vi "cDAQ_Read.vi"(8 "error in":errorcluster, 9 "Prev Temp":dbl format="%0.2f", 10 "DAQ/Control":u16(ring) items=["DAQ", "Control"], 11 "DataCluster":T1={"Core"={"Current VI Reference"=refnum, "Close Panel on Exit?"=FALSE, "Exit"=FALSE}, "Connections"={"cDAQ Therm"={"Task"="", "Connected"=FALSE, "Active"=FALSE}, "cDAQ Voltage"={"Task"="", "Connected"=FALSE, "Active"=FALSE}, "Camera"={"Session"="", "Connected"=FALSE, "Active"=FALSE}}, "Data Acquisition"={"Setup"={"Label"="", "Operator"="", "Notes"="", "TempGrad"=1.0, "TargetTemp"=1.0, "Sample Volume"=1.0}, "Camera"={"Image"=refnum, "Save Image"=refnum, "Image Frequency"=20}, "Thermistor"={"Sample Size"=1, "Calibration"={"B0.100"=[], "R25"=[], "c"=[], "State"=[], "V_S"=5.0, "R_S"=100.0}, "Timing Mode"=14713}, "Partition"={"Data"=[], "Cell Label"="", "Cell Color"=0, "Height"=10, "Width"=16, "Grid"=[]}, "Queue"={"Size"=1, "Queue"=refnum}, "Sample Rate"=1, "Active"=FALSE, "Ready"=FALSE, "Graph Mode"=0}, "Control"={"Sample Rate"=1, "PID gains"={"proportional gain (Kc)"=1.0, "integral time (Ti, min)"=0.01, "derivative time (Td, min)"=0.0}}} {"Control"."PID gains"."derivative time (Td, min)" format="%.3f"; "Control"."PID gains"."integral time (Ti, min)" format="%.3f"; "Control"."PID gains"."proportional gain (Kc)" format="%.3f"; "Control"."Sample Rate" min=1 max=20 step=1 format="%.0f Samples/sec"; "Data Acquisition"."Graph Mode" items=["Average Temperature", "Individual Temperatures"]; "Data Acquisition"."Thermistor"."Timing Mode" items=["Automatic"=16097, "High Resolution"=10195, "High Speed"=14712, "Best 50 Hz Rejection"=14713, "Best 60 Hz Rejection"=14714, "Custom"=10137]; "Data Acquisition"."Thermistor"."Calibration"."R_S" min=0.1 max=1000.0 format="%#_g kOhm"; "Data Acquisition"."Thermistor"."Calibration"."V_S" min=5.0 max=48.0 format="%#_g V"; "Data Acquisition"."Thermistor"."Calibration"."R25" min=0.1 max=1000.0 format="%#_g kOhm"; "Data Acquisition"."Thermistor"."Calibration"."B0.100" min=100.0 max=10000.0 format="%#_g K"; "Data Acquisition"."Thermistor"."Sample Size" min=1 max=200; "Data Acquisition"."Sample Rate" min=20 max=240 format="%.0f samples/min"; "Data Acquisition"."Queue"."Size" min=1 max=200; "Data Acquisition"."Camera"."Image Frequency" min=1 max=60 step=1; "Data Acquisition"."Setup"."Sample Volume" min=0.0 max=500.0 format="%#_g µL"; "Data Acquisition"."Setup"."TargetTemp" min=-40.0 max=40.0 step=0.5 format="%#_g °C"; "Data Acquisition"."Setup"."TempGrad" min=-100.0 max=100.0 step=0.1 format="%#_g °C/min"}) -> (0 "Temp Gradient":dbl, 1 "Mean Temperature":dbl format="%0.2f", 2 "Temperature Readings":dbl[](array[numeric]), 3 "Voltage Readings":dbl[](array[numeric]), 4 "error out":errorcluster, 5 "valid sample?":bool)   [LabVIEW 2020]
uses:
  DataCluster.ctl
  <vilib>/userdefined/High Color/IMAQdx.ctl
  <vilib>/vision/Image Controls.llb/IMAQ Image.ctl
  <vilib>/DAQmx/read.llb/DAQmx Read (Analog 2D DBL NChan NSamp).vi
  <vilib>/Analysis/baseanly.llb/Mean (DBL).vi
  <vilib>/DAQmx/miscellaneous.llb/DAQmx Fill In Error Info.vi
  <vilib>/Analysis/NI_AALBase.lvlib
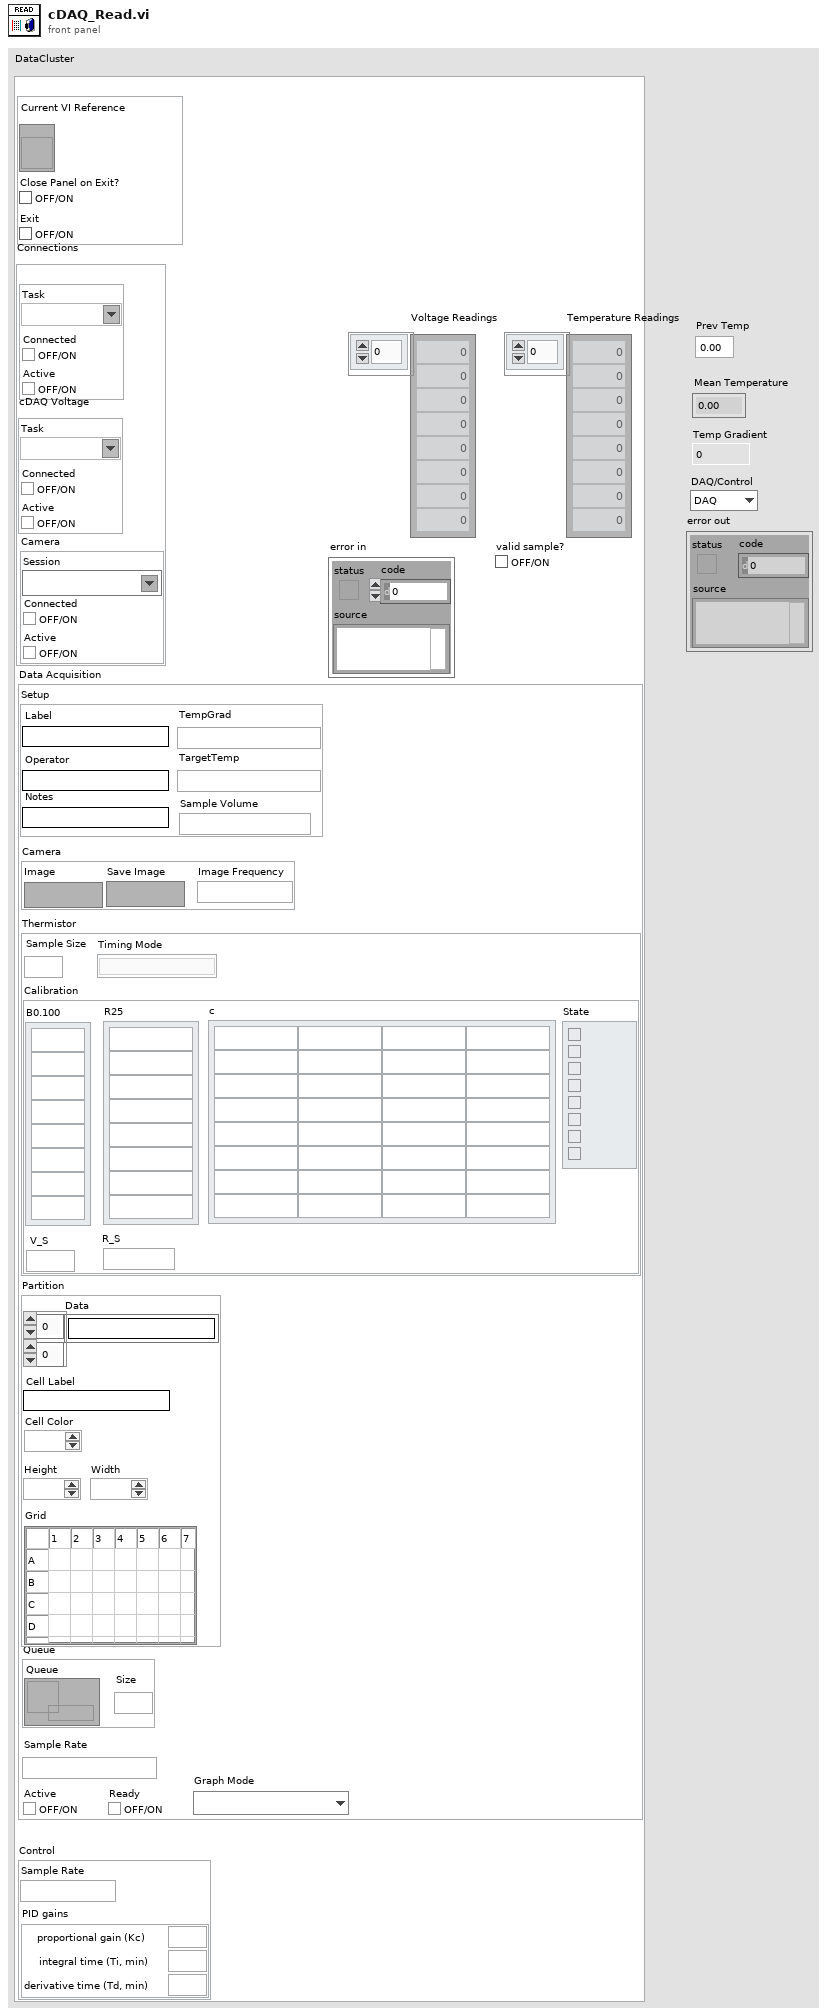
[diagram p1: front panel]
types:
  T1 = typedef "DataCluster.ctl" = cluster{"Core":cluster{"Current VI Reference":refnum<vi>, "Close Panel on Exit?":bool, "Exit":bool}, "Connections":cluster{"cDAQ Therm":cluster{"Task":refnum<k21>, "Connected":bool, "Active":bool}, "cDAQ Voltage":cluster{"Task":refnum<k21>, "Connected":bool, "Active":bool}, "Camera":cluster{"Session":T2, "Connected":bool, "Active":bool}}, "Data Acquisition":cluster{"Setup":cluster{"Label":string, "Operator":string, "Notes":string, "TempGrad":dbl, "TargetTemp":dbl, "Sample Volume":dbl}, "Camera":cluster{"Image":T3, "Save Image":T3, "Image Frequency":i32}, "Thermistor":cluster{"Sample Size":i32, "Calibration":cluster{"B0.100":dbl[], "R25":dbl[], "c":dbl[][], "State":bool[], "V_S":dbl, "R_S":dbl}, "Timing Mode":i32}, "Partition":cluster{"Data":string[][], "Cell Label":string, "Cell Color":u32, "Height":i32, "Width":i32, "Grid":string[][]}, "Queue":cluster{"Size":i32, "Queue":refnum<queue>}, "Sample Rate":i32, "Active":bool, "Ready":bool, "Graph Mode":u16}, "Control":cluster{"Sample Rate":i32, "PID gains":cluster{"proportional gain (Kc)":dbl, "integral time (Ti, min)":dbl, "derivative time (Td, min)":dbl}}}
  T2 = typedef "IMAQdx.ctl" = refnum<k21>
  T3 = typedef "IMAQ Image.ctl" = refnum<image>
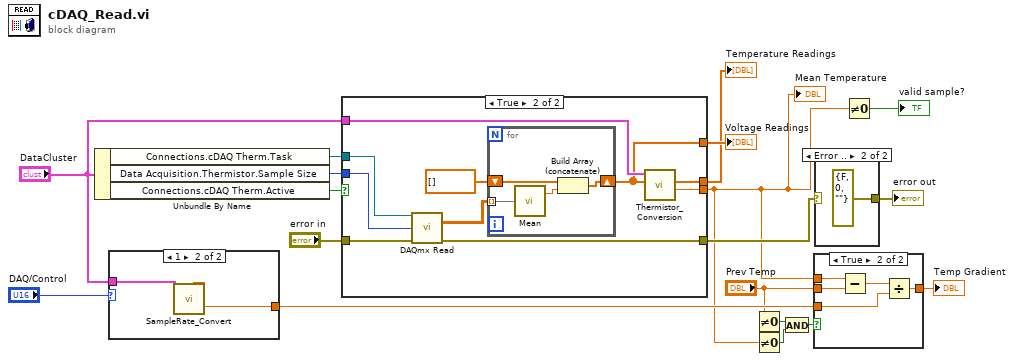
[diagram p0: block diagram]
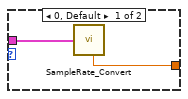
[diagram p4: hidden frame]
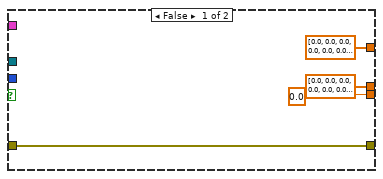
[diagram p5: hidden frame]
diagram:
  n1 = Unbundle By Name("DataCluster") -> ("Connections.cDAQ Therm.Task"=w18:refnum<k21>, "Data Acquisition.Thermistor.Sample Size"=w17:i32, "Connections.cDAQ Therm.Active"=w16:bool)
  n2 = case shown="1" "DAQ/Control" {
    tunnel: [w19 w22] -> w12
    tunnel: "DataCluster" -> [w20 w21]
    frame 0, Default {
      n3 = call "SampleRate_Convert.vi"("DataCluster"=w20) -> ("Sample dt (s)"=w19:dbl)  [unwired: 5 in, 3 out]
    }
    frame 1 {
      n4 = call "SampleRate_Convert.vi"("DataCluster"=w21) -> ("Control Sample dt (s)"=w22:dbl)  [unwired: 5 in, 3 out]
    }
  }
  n5 = case shown="True" w16 {
    tunnel: w18 -> [_ w36]
    tunnel: [dbl[] [0.0, 0.0, 0.0, 0.0, 0.0, 0.0, 0.0, 0.0] w31] -> w15
    tunnel: w17 -> [_ w33]
    tunnel: "DataCluster" -> [_ w32]
    tunnel: [dbl[] [0.0, 0.0, 0.0, 0.0, 0.0, 0.0, 0.0, 0.0] ("Temperature Readings") w30] -> w14
    tunnel: "error in" -> [w24 w29]
    tunnel: [w24 w28] -> w7
    tunnel: [0.0 ("Mean Temp") w27] -> w1
    frame False {
    }
    frame True {
      n6 = call-poly <vilib>:"DAQmx Read.vi"("task/channels in"=w36, "number of samples per channel"=w33, "error in"=w29) -> ("data"=w35:dbl[][], "error out"=w28:errorcluster)  [unwired: 10 in, 1 out]
      n7 = for {
        tunnel: w35 -> [w40] mode=indexing
        shift-right: [w39] -> w31
        shift-left: dbl[] [] -> [w38]
        n8 = call-poly <vilib>:"Mean.vi"("X"=w40) -> ("mean"=w37:dbl)  [unwired: 1 out]
        n9 = Build Array (concatenate)(w38, w37) -> (w39:dbl[])
      }
      n10 = call "Thermistor_Conversion.vi"("Voltage Readings"=w31, "DataCluster"=w32) -> ("Mean Temp"=w27:dbl, "Temperature Readings"=w30:dbl[])  [unwired: 8 in]
    }
  }
  "Voltage Readings" <- w15
  "Temperature Readings" <- w14
  "Mean Temperature" <- w1
  n11 = Not Equal To 0?(x="Prev Temp") -> (x != 0?=w5:bool)
  n12 = Not Equal To 0?(x=w1) -> (x != 0?=w2:bool)
  n13 = And(x=w5, y=w2) -> (x .and. y?=w3:bool)
  n14 = case shown="True" w3 {
    tunnel: "Prev Temp" -> [_ w44]
    tunnel: w12 -> [_ w43]
    tunnel: [_ w42] -> w10
    tunnel: w1 -> [_ w41]
    frame False {
    }
    frame True {
      n15 = Subtract(x=w41, y=w44) -> (x-y=w45:dbl)
      n16 = Divide(x=w45, y=w43) -> (x/y=w42:dbl)
    }
  }
  "Temp Gradient" <- w10
  n17 = case shown="Error .." w7 {
    selector: w7 -> [w46 _]
    tunnel: [w46 errorcluster {"status"=FALSE, "code"=0, "source"=""} ("error IO")] -> w8
    frame No Error {
    }
    frame Error {
    }
  }
  "error out" <- w8
  n18 = Not Equal To 0?(x=w1) -> (x != 0?=→"valid sample?":bool)
